vi "SMTP Email Send Message.vi"(0 "recipients":string[](array[string]), 1 "mail server":string, 2 "return address":string, 5 "subject ([No Subject])":string="[No Subject]", 7 "message":string, 11 "error in (no error)":errorcluster, 12 "username":string, 13 "password":string) -> (4 "invalid recipients":string[](array[string]), 15 "error out":errorcluster)   [LabVIEW 2011, in "NewNI_SMTPEmail.lvlib"]
doc: "Sends a text email to a list of recipients."
uses:
  NewNI_SMTPEmail.lvlib
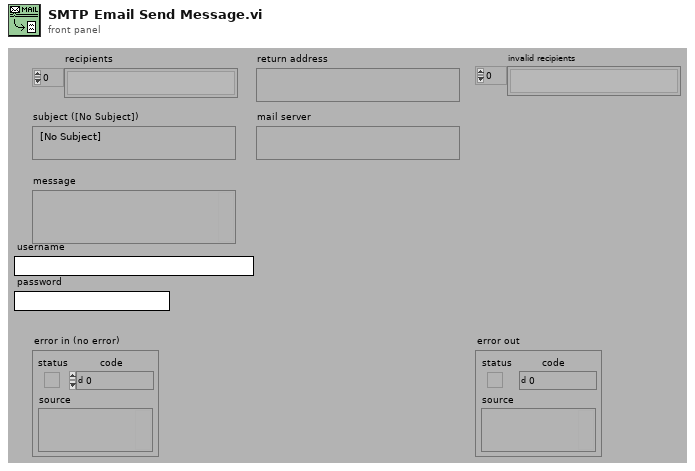
[diagram p1: front panel]
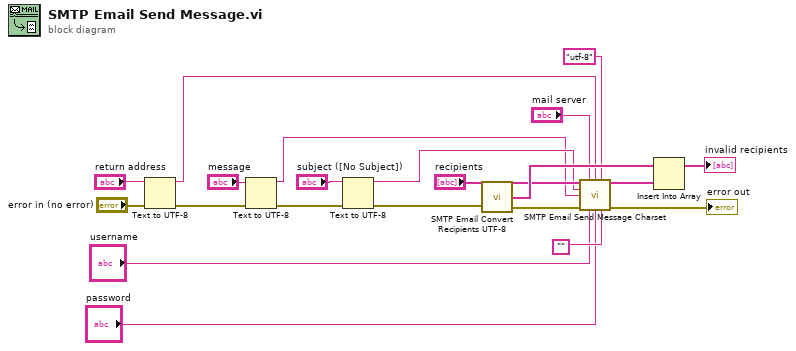
[diagram p0: block diagram]
diagram:
  n1 = Text to UTF-8(8:"error in (no error)", 11:"return address") -> (0:w16:errorcluster, 3:w7:string)
  n2 = Text to UTF-8(8:w16, 11:"message") -> (0:w17:errorcluster, 3:w8:string)
  n3 = Text to UTF-8(8:w17, 11:"subject ([No Subject])") -> (0:w14:errorcluster, 3:w9:string)
  n4 = call "SMTP Email Convert Recipients UTF-8.vi"("recipients"="recipients", "error in"=w14) -> ("convertible recipients"=w10:string[], "unconvertible recipients"=w12:string[], "error out"=w4:errorcluster)
  n5 = call "SMTP Email Send Message Charset.vi"("recipients"=w10, "mail server"="mail server", "return address"=w7, "character set (us-ascii)"="utf-8", "subject ([No Subject])"=w9, "message"=w8, "error in (no error)"=w4, "username"="username", "password"="password", "translit"="") -> ("invalid recipients"=w13:string[], "error out"=→"error out":errorcluster)  [unwired: 4 out]
  n6 = Insert Into Array(array=w12, new element=w13) -> (→"invalid recipients":string[])  [unwired: 1 in]
